vi "FTW-Test-Regex-BasicUsage.vi"() -> (0 "Test Result":errorcluster)   [LabVIEW 2014]
uses:
  src/error/FTW-ERR-ThrowInfo.vi
  src/error/FTW-ERR-ThrowError.vi
  src/error/FTW-ERR-CallChain.vi
  src/string/FTW-STR-ReplaceWhitespace.vi
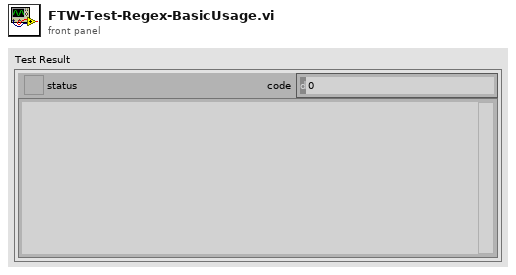
[diagram p1: front panel]
types:
  T1 = cluster{"callout_id":i32, "subject_current_pos":i32, "subject_start_match_pos":i32, "cap_top":i32, "cap_last":i32, "patt_pos":i32, "callout_name_index":i32, "callout_name_length":i32}[]
  T2 = cluster{"callout_id":i32, "subject_current_pos":i32, "subject_start_match_pos":i32, "cap_top":i32, "cap_last":i32, "patt_pos":i32, "callout_name_index":i32, "callout_name_length":i32}
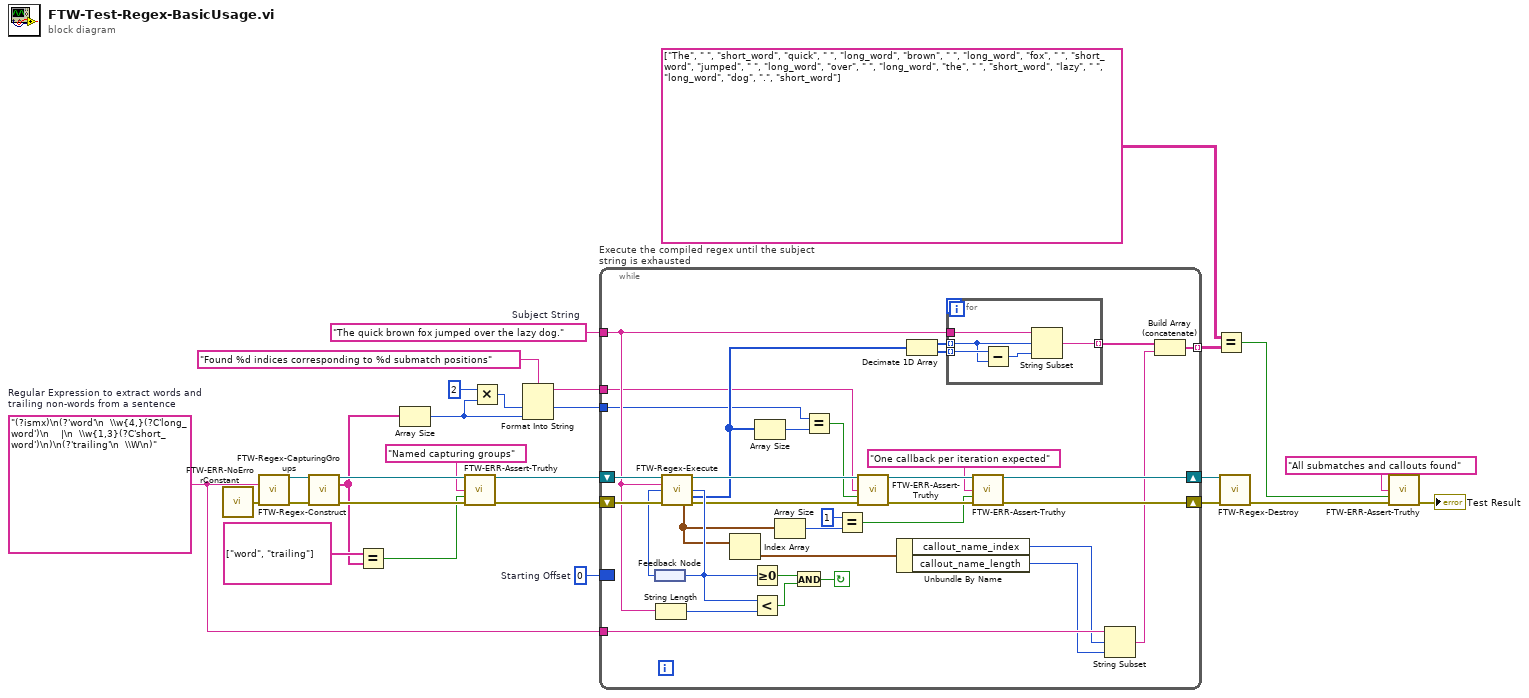
[diagram p0: block diagram]
diagram:
  w1 = "(?ismx)\n(?'word'\n  \\w{4,}(?C'long_word')\n    |\n  \\w{1,3}(?C'short_word')\n)\n(?'trailing'\n  \\W\n)"  # Regular Expression to extract words and trailing non-words from a sentence
  w17 = 0  # Starting Offset
  w18 = "The quick brown fox jumped over the lazy dog."  # Subject String
  n1 = call "FTW-ERR-NoErrorConstant.vi"() -> ("no error"=w23:errorcluster)
  n2 = call "FTW-Regex-Construct.vi"("Regular Expression"=w1, "error in"=w23) -> ("Regex"=w25:refnum<data-value>, "error out"=w24:errorcluster)  [unwired: 12 in]
  n3 = call "FTW-Regex-CapturingGroups.vi"("Regex"=w25, "error in"=w24) -> ("Regex out"=w22:refnum<data-value>, "Capture Groups"=w7:string[], "error out"=w12:errorcluster)  [unwired: 11 in]
  n4 = Equal?(x=string[] ["word", "trailing"], y=w7) -> (x = y?=w10:bool)
  n5 = Array Size(array=w7) -> (size(s)=w6:i32)
  n6 = call "FTW-ERR-Assert-Truthy.vi"("Assertion"="Named capturing groups", "Assertion holds true?"=w10, "error in"=w12) -> ("error out"=w11:errorcluster)  [unwired: 12 in]
  n7 = Multiply(x=2, y=w6) -> (x*y=w3:i32)
  n8 = Format Into String(format string="Found %d indices corresponding to %d submatch positions" ("Assertion"), w3, w6) -> (resulting string=w2:string)  [unwired: 2 in, 1 out]
  n9 = while "Execute the compiled regex until the subject string is exhausted" {
    shift-right: [w57] -> w21
    shift-left: w22 -> [w58]
    shift-right: [w39] -> w20
    shift-left: w11 -> [w56]
    tunnel: w18 -> [w54]
    tunnel: [w27] -> w16 mode=indexing
    border: w17 -> [_]
    tunnel: w3 -> [w42]
    tunnel: w2 -> [w41]
    tunnel: w1 -> [w32]
    stop <- w49 continue-if-true
    n10 = feedback #1() -> (w55:i32)
    n11 = String Length(string=w54) -> (length=w52:i32)
    n12 = call "FTW-Regex-Execute.vi"("Regex"=w58, "Subject String"=w54, "Starting Offset"=w55, "error in"=w56) -> ("Regex out"=w57:refnum<data-value>, "Offset after Match"=w53:i32, "Submatches"=w45:i32[], "Callouts"=w34:T1, "error out"=w46:errorcluster)  [unwired: 6 in, 1 out]
    n13 = feedback-in #1(w53) -> ()
    n14 = Index Array(array=w34) -> (element=w33:T2)  [unwired: 1 in]
    n15 = Greater Or Equal To 0?(x=w53) -> (x >= 0?=w50:bool)
    n16 = Less?(x=w53, y=w52) -> (x < y?=w51:bool)
    n17 = Array Size(array=w45) -> (size(s)=w44:i32)
    n18 = Array Size(array=w34) -> (size(s)=w38:i32)
    n19 = And(x=w50, y=w51) -> (x .and. y?=w49:bool)
    n20 = Equal?(x=w42, y=w44) -> (x = y?=w43:bool)
    n21 = Equal?(x=1, y=w38) -> (x = y?=w36:bool)
    n22 = call "FTW-ERR-Assert-Truthy.vi"("Assertion"=w41, "Assertion holds true?"=w43, "error in"=w46) -> ("error out"=w40:errorcluster)  [unwired: 12 in]
    n23 = Unbundle By Name(w33) -> ("callout_name_index"=w31:i32, "callout_name_length"=w30:i32)
    n24 = Decimate 1D Array(w45) -> (w48:i32[], w47:i32[])
    n25 = for {
      tunnel: w47 -> [w62] mode=indexing
      tunnel: w48 -> [w61] mode=indexing
      tunnel: w54 -> [w63]
      tunnel: [w59] -> w29 mode=indexing
      n26 = Subtract(x=w62, y=w61) -> (x-y=w60:i32)
      n27 = String Subset(string=w63, offset (0)=w61, length (rest)=w60) -> (substring=w59:string)
    }
    n28 = call "FTW-ERR-Assert-Truthy.vi"("Assertion"="One callback per iteration expected", "Assertion holds true?"=w36, "error in"=w40) -> ("error out"=w39:errorcluster)  [unwired: 12 in]
    n29 = String Subset(string=w32, offset (0)=w31, length (rest)=w30) -> (substring=w28:string)
    n30 = Build Array (concatenate)(w29, w28) -> (w27:string[])
  }
  n31 = Equal?(x=string[][] [["The", " ", "short_word"], ["quick", " ", "long_word"], ["brown", " ", "long_word"], ["fox", " ", "short_word"], ["jumped", " ", "long_word"], ["over", " ", "long_word"], ["the", " ", "short_word"], ["lazy", " ", "long_word"], ["dog", ".", "short_word"]] ("Array 2"), y=w16) -> (x = y?=w15:bool)
  n32 = call "FTW-Regex-Destroy.vi"("Regex"=w21, "error in"=w20) -> ("error out"=w19:errorcluster)  [unwired: 13 in]
  n33 = call "FTW-ERR-Assert-Truthy.vi"("Assertion"="All submatches and callouts found", "Assertion holds true?"=w15, "error in"=w19) -> ("error out"=→"Test Result":errorcluster)  [unwired: 12 in]
